vi "Asylum_GetValue.vi"(8 "error in (no error)":errorcluster, 10 "Value":string, 11 "Application":refnum<k7>) -> (0 "error out":errorcluster, 2 "Value":dbl, 3 "Application":refnum<k7>)   [LabVIEW 2019]
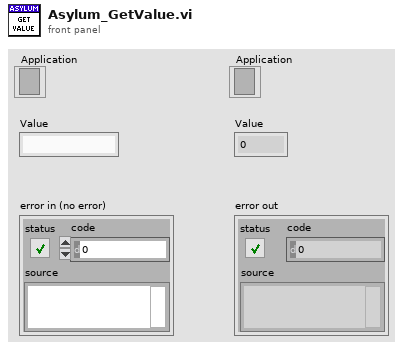
[diagram p1: front panel]
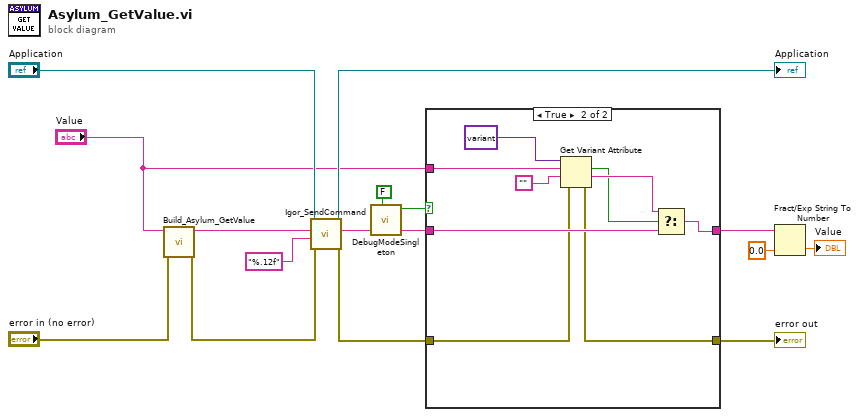
[diagram p0: block diagram]
diagram:
  n1 = call "Build_Asylum_GetValue.vi"("error in (no error)"="error in (no error)", "Value"="Value") -> ("error out"=w2:errorcluster, "String"=w3:string)  [unwired: 8 in]
  n2 = call <userlib>:"Igor_SendCommand.vi"("error in (no error)"=w2, "Format"="%.12f" ("Expected output Format"), "command"=w3, "Application In"="Application") -> ("error out"=w6:errorcluster, "results"=w10:string, "Application Out"=→"Application":refnum<k7>)  [unwired: 4 in, 1 out]
  n3 = call <userlib>:"DebugModeSingleton.vi"("Write?"=FALSE) -> ("Debug Mode?"=w8:bool)  [unwired: 10 in]
  n4 = case shown="True" w8 {
    tunnel: w10 -> [w17 w22]
    tunnel: [w17 w23] -> w9
    tunnel: "Value" -> [_ w26]
    tunnel: w6 -> [w16 w18]
    tunnel: [w16 w19] -> w5
    frame False {
    }
    frame True {
      n5 = Get Variant Attribute(Variant=variant variant ("Notes LUT"), name=w26, default value (empty Variant)="", error in=w18) -> (names=w21:bool, values=w24:string, error out=w19:errorcluster)  [unwired: 1 out]
      n6 = Select(t=w24, s=w21, f=w22) -> (s? t:f=w23:string)
    }
  }
  "error out" <- w5
  n7 = Fract/Exp String To Number(string=w9, default (0 dbl)=0.0 ("default (0 DBL)")) -> (number=→"Value":dbl)  [unwired: 3 out]
